vi "toml_api_get.vi"(6 "default":variant, 7 "resolved path":path, 8 "error in (no error)":errorcluster, 9 "key":string, 10 "section":string, 11 "vi in":refnum<vi>) -> (0 "error out":errorcluster, 1 "value":variant, 2 "key exists":bool, 3 "vi out":refnum<vi>)   [LabVIEW 2017]
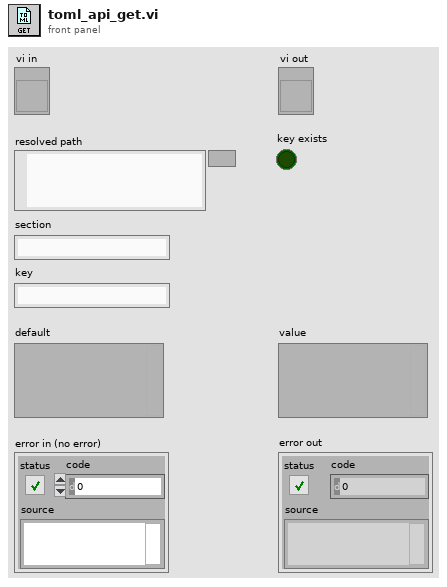
[diagram p1: front panel]
types:
  T1 = cluster{"section":string, "key":string, "default":variant}
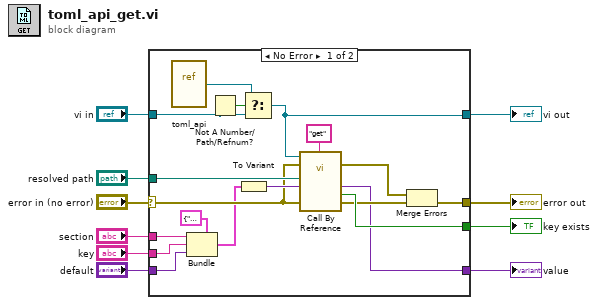
[diagram p0: block diagram]
diagram:
  n1 = case shown="No Error" "error in (no error)" {
    selector: "error in (no error)" -> [w19 w31]
    tunnel: [w27 _] -> w10
    tunnel: "resolved path" -> [w25 _]
    tunnel: [w21 w31] -> w8
    tunnel: "vi in" -> [w18 w30]
    tunnel: [w17 w30] -> w5
    tunnel: "section" -> [w16 _]
    tunnel: "key" -> [w15 _]
    tunnel: "default" -> [w14 w29]
    tunnel: [w11 w29] -> w1
    frame No Error {
      n2 = vi-ref "toml_api.vi"() -> (w24:refnum<vi>)
      n3 = Bundle(cluster=T1 {"section"="", "key"="", "default"=variant}, "section"=w16, "key"=w15, "default"=w14) -> (w13:T1)
      n4 = Not A Number/Path/Refnum?(number/path/refnum=w18) -> (NaN/Path/Refnum?=w23:bool)
      n5 = To Variant(anything=w13) -> (Variant=w28:variant)
      n6 = Select(t=w24, s=w23, f=w18) -> (s? t:f=w17:refnum<vi>)
      n7 = call-by-ref "?"(reference=w17, error in=w19, "cmd"="get", 8:"error in (no error)"=w19, "data in"=w28, "path in"=w25) -> (error out=w20:errorcluster, 0:"error out"=w26:errorcluster, "return"=w27:bool, "data out"=w11:variant)  [unwired: 4 in, 2 out]
      n8 = Merge Errors(w20, w26) -> (w21:errorcluster)
    }
    frame Error {
    }
  }
  "key exists" <- w10
  "error out" <- w8
  "vi out" <- w5
  "value" <- w1
